vi "build_name.vi"(4 "error in":errorcluster, 6 "Configuration":string, 7 "Name":string) -> (0 "error out":errorcluster, 2 "Name":string, 3 "Type":string)   [LabVIEW 2019]
doc: "Builds the name of a file based on the type of sensor and the custom name the user provided."
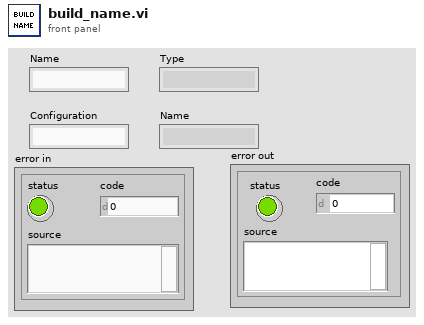
[diagram p1: front panel]
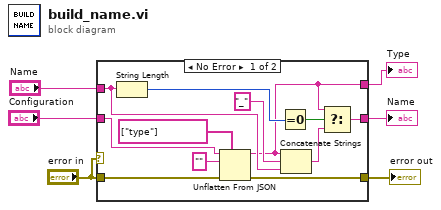
[diagram p0: block diagram]
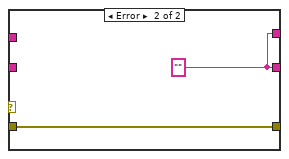
[diagram p2: hidden frame]
diagram:
  n1 = case shown="No Error" "error in" {
    tunnel: "error in" -> [w12 w20]
    tunnel: [w11 w20] -> w5
    tunnel: "Name" -> [w10 _]
    tunnel: "Configuration" -> [w9 _]
    tunnel: [w8 w19] -> w2
    tunnel: [w7 w19] -> w1
    frame No Error {
      n2 = String Length(string=w10) -> (length=w13:i32)
      n3 = Unflatten From JSON(path=string[] ["type"], JSON string=w9, type and defaults="", error in (no error)=w12) -> (value=w7:string, error out=w11:errorcluster)  [unwired: 3 in]
      n4 = Equal To 0?(x=w13) -> (x = 0?=w14:bool)
      n5 = Concatenate Strings(w7, "_" ("string"), w10) -> (w15:string)
      n6 = Select(t=w7, s=w14, f=w15) -> (s? t:f=w8:string)
    }
    frame Error {
      w19 = ""
    }
  }
  "error out" <- w5
  "Name" <- w2
  "Type" <- w1
